vi "Get Mode Index.vi"(8 "error in (no error)":errorcluster, 11 "Pulseblaster in":refnum<class "Pulseblaster.lvclass">) -> (0 "error out":errorcluster, 2 "Mode Col":i32, 3 "Pulseblaster out":refnum<class "Pulseblaster.lvclass">)   [LabVIEW 2013, in "Pulseblaster.lvclass"]
uses:
  Pulseblaster.lvclass
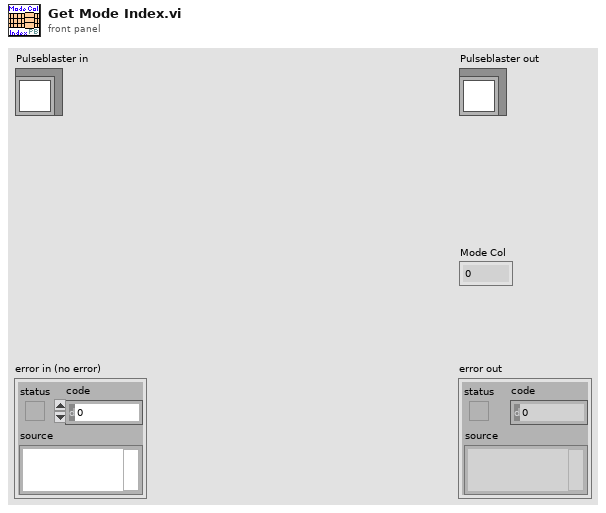
[diagram p1: front panel]
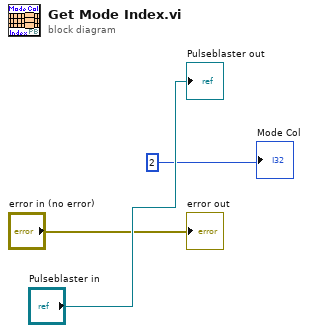
[diagram p0: block diagram]
diagram:
  "error out" <- "error in (no error)"
  "Pulseblaster out" <- "Pulseblaster in"
  "Mode Col" <- 2 ("Mode Col")
